vi "Launch Module.vi"(8 "error in":errorcluster) -> (0 "error out":errorcluster)   [LabVIEW 2023, in "Adjust FP VIs.lvlib"]
uses:
  _Adjust FP VIs/Adjust FP VIs.lvlib
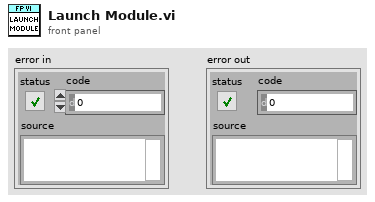
[diagram p1: front panel]
types:
  T1 = enum32{"Invalid", "Standard", "Closed", "Hidden", "Minimized", "Maximized"}
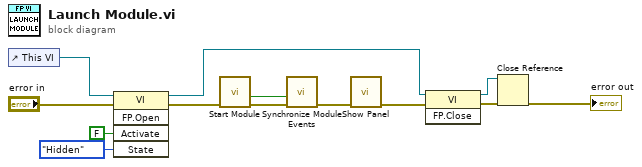
[diagram p0: block diagram]
diagram:
  n1 = control-ref of="This VI"() -> (w11:refnum<vi>)
  n2 = invoke class="VI" method="FP.Open"(reference=w11, error in="error in", "Activate"=FALSE ("Activate?"), "State"=T1."Hidden") -> (reference out=w6:refnum<vi>, error out=w7:errorcluster)  [unwired: 1 in, 3 out]
  n3 = call "Start Module.vi"("error in"=w7) -> ("error out"=w12:errorcluster, "Wait for Event Sync?"=w13:bool)  [unwired: 6 in, 3 out]
  n4 = call "Synchronize Module Events.vi"("error in"=w12, "Wait for Event Sync?"=w13) -> ("error out"=w2:errorcluster)  [unwired: 9 in]
  n5 = call "Show Panel.vi"("error in"=w2) -> ("error out"=w1:errorcluster)  [unwired: 10 in]
  n6 = invoke class="VI" method="FP.Close"(reference=w6, error in=w1) -> (reference out=w4:refnum<vi>, error out=w5:errorcluster)  [unwired: 1 in, 1 out]
  n7 = Close Reference(reference=w4, error in (no error)=w5) -> (error out=→"error out":errorcluster)
